vi "Find Outputs in Dictionary.vi"(8 "error in (no error)":errorcluster, 9 "processing data dictionary":refnum<class "data dictionary.lvclass">, 10 "PID Loops":refnum<class "PID Loop.lvclass">[](array[class]), 11 "Tagbus PID Module runtime in":refnum<class "PID Module runtime.lvclass">) -> (0 "error out":errorcluster, 3 "Tagbus PID Module runtime out":refnum<class "PID Module runtime.lvclass">)   [LabVIEW 2014, in "PID Module runtime.lvclass"]
uses:
  PID Module runtime.lvclass
  <vilib>/NI/Tag Bus/dictionary/data dictionary.lvclass
  configuration/PID Loop.lvclass
  <vilib>/NI/Tag Bus/tag/Data Type.ctl
  configuration/PID Loop/String Parameters.ctl
  PID Module runtime.lvclass/PID Module runtime.ctl
  <vilib>/NI/Tag Bus/tag/tag descriptor.lvclass
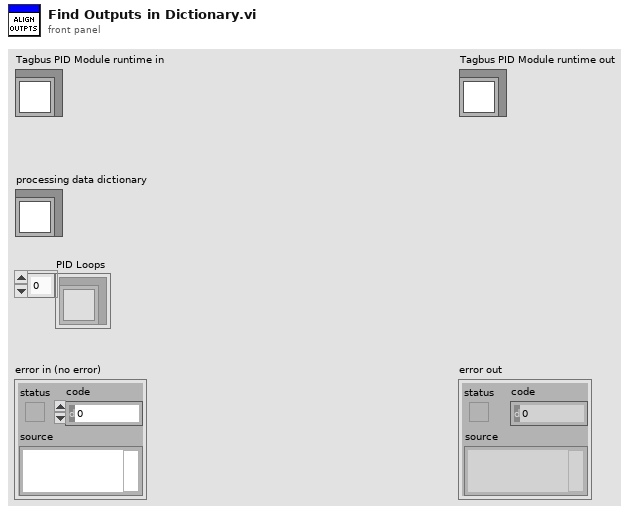
[diagram p1: front panel]
types:
  T1 = typedef "PID Loop.lvclass/String Parameters.ctl" = enum16{"Setpoint", "Process Variable", "Output", "Proportional Gain", "Integral Time", "Derivative Time", "Range High", "Range Low"}
  T2 = typedef "tag bus.lvlib/tag descriptor.lvclass/Data Type.ctl" = enum16{"Double", "Single", "I64", "I32", "I16", "I8", "U64", "U32", "U16", "U8", "Boolean", "String", "Array of Double", "Array of Single", "Array of I64", "Array of I32", "Array of I16", "Array of I8", "Array of U64", "Array of U32", "Array of U16", "Array of U8", "Array of Boolean", "Array of String"}
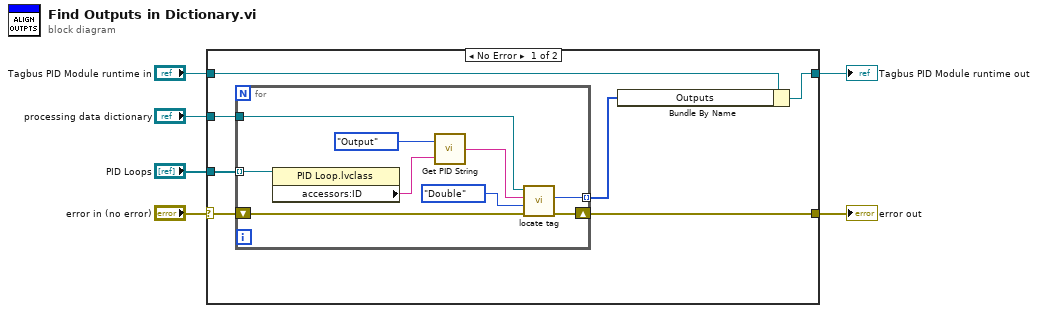
[diagram p0: block diagram]
diagram:
  n1 = case shown="No Error" "error in (no error)" {
    selector: "error in (no error)" -> [w8 w24]
    tunnel: [w7 w24] -> w2
    tunnel: "processing data dictionary" -> [w13 _]
    tunnel: "PID Loops" -> [w12 _]
    tunnel: "Tagbus PID Module runtime in" -> [w11 w23]
    tunnel: [w9 w23] -> w3
    frame No Error {
      n2 = for {
        tunnel: w13 -> [w22]
        tunnel: w12 -> [w17] mode=indexing
        tunnel: [w20] -> w10 mode=indexing
        shift-right: [w18] -> w7
        shift-left: w8 -> [w19]
        n3 = property class="PID Loop.lvclass"(reference=w17) -> ("accessors:ID"=w16:string)  [unwired: 1 in, 2 out]
        n4 = call "Get PID String.vi"("PID Loop ID"=w16, "PID Parameter"=String_Parameters."Output") -> ("Parameter String"=w14:string)
        n5 = call <vilib>:"locate tag.vi"("error in"=w19, "data type"=Data_Type."Double", "name"=w14, "data dictionary in"=w22) -> ("error out"=w18:errorcluster, "index"=w20:i32)  [unwired: 5 in, 1 out]
      }
      n6 = Bundle By Name(cluster=w11, "Outputs"=w10) -> (w9:refnum<class "PID Module runtime.lvclass">)
    }
    frame Error {
    }
  }
  "error out" <- w2
  "Tagbus PID Module runtime out" <- w3
